vi "PH_SystemInformation.ProcCases.vi"(0 "i ref in":refnum<vi>, 1 "selector":string, 2 "Data":T1, 3 "call cluster":T2={"Object"="", "Selector"="", "CallType"=enum."synchronous", "Async Object"="", "Async Selector"="", "Data Descriptor"="", "Data"=[], "Error #"=0, "Expire"=0}, 5 "error in (no error)":errorcluster) -> (14 "i ref out":refnum<vi>, 17 "answer cluster":T2={"Object"="", "Selector"="", "CallType"=enum."synchronous", "Async Object"="", "Async Selector"="", "Data Descriptor"="", "Data"=[], "Error #"=0, "Expire"=0}, 19 "error out":errorcluster)   [LabVIEW 2014, in "PH_SystemInformation.lvlib"]
doc: "This method is called by a process from within the default case in the event loop. The methods of a class that are linked to events will be called from THIS method. Add your code here."
uses:
  PH_SystemInformation.lvlib
  CS_Core/CSSystem/CoreDefs/CoreDefs.call_type.ctl
  CS_Core/BaseProcess/BaseProcess.descriptor string definition.ctl
  CS_Core/CSSystem/CoreDefs/CoreDefs.rawDataType.ctl
  PH_SystemInformationEnabling State.ctl
  CS_Core/CSSystem/CoreLib/CoreLib.string 2 byte array.vi
  CS_Core/BaseProcess/BaseProcess.lvlib
  PH_Common/PH_Common.lvlib
  CS_Core/CAEObj/CAEObj.lvlib
  CS_Core/CSSystem/CoreLib/CoreLib.lvlib
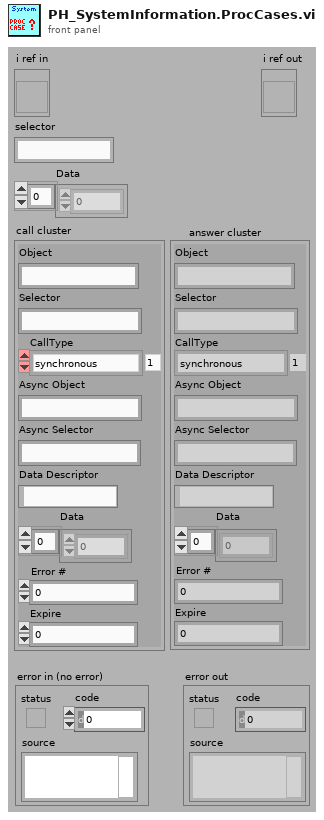
[diagram p1: front panel]
types:
  T1 = typedef "CoreDefs.rawDataType.ctl" = i8[]
  T2 = typedef "CoreDefs.call_type.ctl" = cluster{"Object":string, "Selector":string, "CallType":enum16{"simple", "synchronous", "asynchronous"}, "Async Object":string, "Async Selector":string, "Data Descriptor":T3, "Data":T1, "Error #":i32, "Expire":u32}
  T3 = typedef "BaseProcess.lvlib/BaseProcess.descriptor string definition.ctl" = string
  T4 = typedef "PH_SystemInformation.lvlib/PH_SystemInformation.i attribute.ctl" = cluster{"Laser Enabling":cluster{"GUI Ref":refnum<vi>, "Enabling State":T5}, "PreAmp Enabling":cluster{"GUI Ref":refnum<vi>, "Enabling State":T5}, "MainAmp Enabling":cluster{"GUI Ref":refnum<vi>, "Enabling State":T5}, "Emergency Off":cluster{"GUI Ref":refnum<vi>, "State":enum16{"no info", "off/false", "Alarm"}}, "Enabling Exp. 1":cluster{"GUI Ref":refnum<vi>, "Enabling State":T5}, "Enabling Exp. 2":cluster{"GUI Ref":refnum<vi>, "Enabling State":T5}, "Enabling Exp. 3":cluster{"GUI Ref":refnum<vi>, "Enabling State":T5}, "Enabling Exp. 4":cluster{"GUI Ref":refnum<vi>, "Enabling State":T5}, "Timing Mode":cluster{"GUI Ref":refnum<vi>, "PHELIX_Timing_Mode":enum32{"10 Hz", "0.5 Hz", "Shot"}}}
  T5 = typedef "PH_SystemInformation.lvlib/PH_SystemInformationEnabling State.ctl" = i32
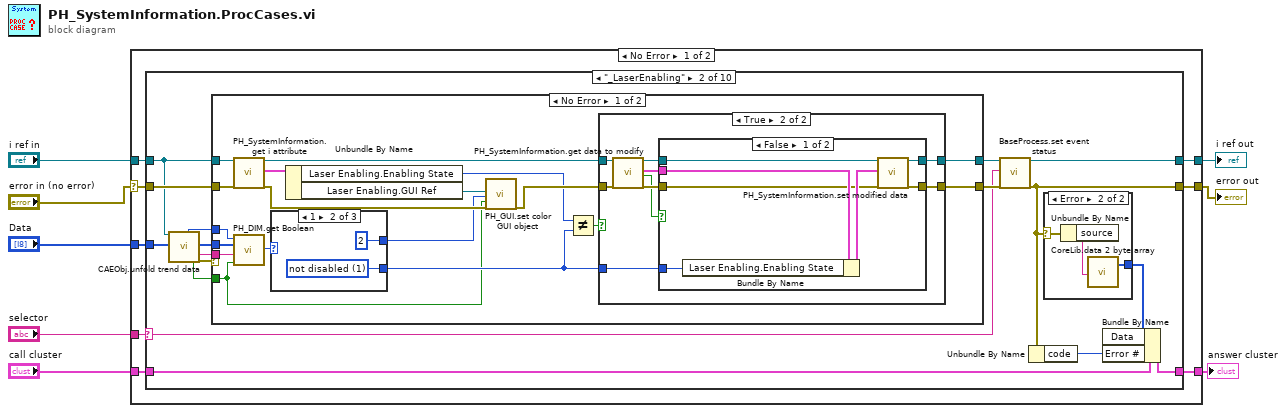
[diagram p0: block diagram]
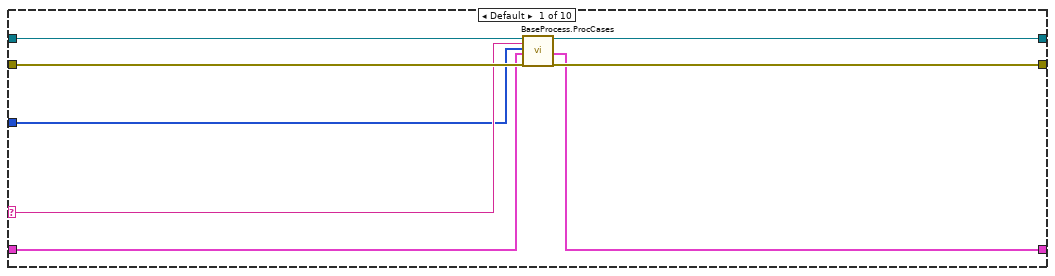
[diagram p2: hidden frame]
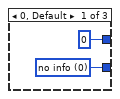
[diagram p6: hidden frame]
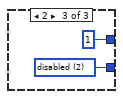
[diagram p7: hidden frame]
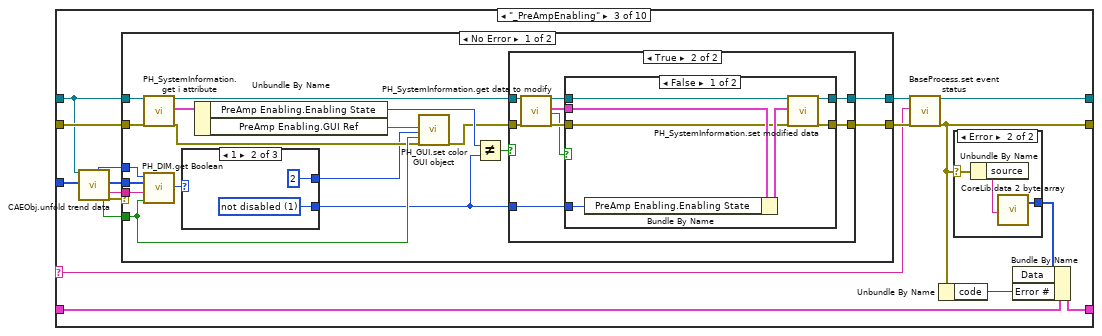
[diagram p9: hidden frame]
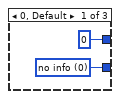
[diagram p13: hidden frame]
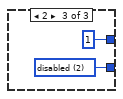
[diagram p14: hidden frame]
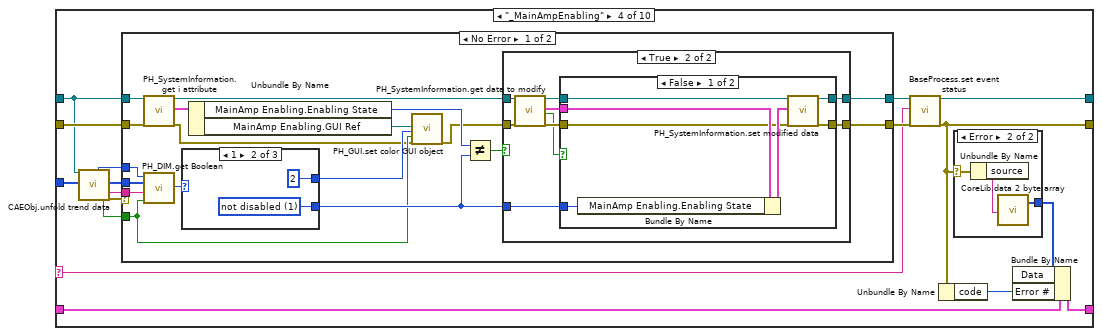
[diagram p16: hidden frame]
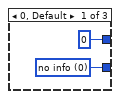
[diagram p20: hidden frame]
diagram:
  n1 = case shown="No Error" "error in (no error)" {
    selector: "error in (no error)" -> [w9 w624]
    tunnel: "selector" -> [w16 _]
    tunnel: [w15 w623] -> w7
    tunnel: "call cluster" -> [w14 w623]
    tunnel: "i ref in" -> [w13 w625]
    tunnel: [w12 w625] -> w4
    tunnel: [w11 w624] -> w3
    tunnel: "Data" -> [w10 _]
    frame No Error {
      n2 = case shown="\"_LaserEnabling\"" w16 {
        selector: w16 -> [w19 w27 w93 w159 w225 w291 w357 w423 w489 w555]
        tunnel: w10 -> [w17 w40 w106 w172 w238 w304 w370 w436 w502 w566]
        tunnel: w13 -> [w18 w39 w105 w171 w237 w303 w369 w435 w501 w565]
        tunnel: [w24 w28 w94 w160 w226 w292 w358 w424 w490 w556] -> w12
        tunnel: w14 -> [w20 w26 w92 w158 w224 w290 w356 w422 w488 w554]
        tunnel: [w21 w25 w91 w157 w223 w289 w355 w421 w487 w553] -> w15
        tunnel: w9 -> [w23 w41 w107 w173 w239 w305 w371 w437 w503 w567]
        tunnel: [w22 w29 w95 w161 w227 w293 w359 w425 w491 w557] -> w11
        frame Default {
          n3 = call "BaseProcess.ProcCases.vi"("i ref in"=w18, "selector"=w19, "Data"=w17, "call cluster"=w20, "error in (no error)"=w23) -> ("i ref out"=w24:refnum<vi>, "answer cluster"=w21:T2, "error out"=w22:errorcluster)  [unwired: 12 in]
        }
        frame "_LaserEnabling" {
          n4 = call "CAEObj.unfold trend data.vi"("i ref in"=w39, "raw trend data"=w40) -> ("quality"=w38:i32, "no link"=w36:bool, "data"=w35:i8[], "typeDescriptor"=w37:string, "error out"=w34:errorcluster)  [unwired: 9 in, 4 out]
          n5 = case shown="No Error" w34 {
            tunnel: [w57 w90] -> w30
            tunnel: w39 -> [w56 w90]
            tunnel: w41 -> [w62 w89]
            tunnel: [w58 w89] -> w31
            tunnel: w38 -> [w61 _]
            tunnel: w37 -> [w60 _]
            tunnel: w36 -> [w46 _]
            tunnel: w35 -> [w59 _]
            frame No Error {
              n6 = call "PH_SystemInformation.get i attribute.vi"("i ref in"=w56, "error in (no error)"=w62) -> ("i ref out"=w55:refnum<vi>, "i attribute"=w53:T4, "error out"=w50:errorcluster)  [unwired: 15 in]
              n7 = call "PH_DIM.get Boolean.vi"("no link"=w46, "typeDescriptor"=w60, "data"=w59, "quality"=w61) -> ("Value"=w54:i32)
              n8 = case shown="1" w54 {
                tunnel: [0 2 1] -> w47
                tunnel: [w83 w85 w87] -> w52
                frame 0, Default {
                  w83 = T5 0 items=["no info", "not disabled", "disabled"] ("Laser Enabling.Enabling State")
                }
                frame 1 {
                  w85 = T5 1 items=["no info", "not disabled", "disabled"] ("Laser Enabling.Enabling State")
                }
                frame 2 {
                  w87 = T5 2 items=["no info", "not disabled", "disabled"] ("Laser Enabling.Enabling State")
                }
              }
              n9 = Unbundle By Name(w53) -> ("Laser Enabling.Enabling State"=w45:T5, "Laser Enabling.GUI Ref"=w48:refnum<vi>)
              n10 = call "PH_GUI.set color GUI object.vi"("GUI object Ref"=w48, "State"=w47, "Blinking? (false)"=w46, "error in (no error)"=w50) -> ("error out"=w49:errorcluster)  [unwired: 15 in]
              n11 = Not Equal?(x=w45, y=w52) -> (x != y?=w51:bool)
              n12 = case shown="True" w51 {
                tunnel: [w63 w71] -> w58
                tunnel: [w64 w69] -> w57
                tunnel: w49 -> [w63 w67]
                tunnel: w55 -> [w64 w66]
                tunnel: w52 -> [_ w65]
                frame False {
                }
                frame True {
                  n13 = call "PH_SystemInformation.get data to modify.vi"("i ref in"=w66, "error in (no error)"=w67) -> ("i ref out"=w70:refnum<vi>, "i attribute"=w72:T4, "timed out"=w68:bool, "error out"=w73:errorcluster)  [unwired: 14 in]
                  n14 = case shown="False" w68 {
                    tunnel: w73 -> [w74 w81]
                    tunnel: w72 -> [w77 _]
                    tunnel: [w80 w81] -> w71
                    tunnel: w70 -> [w79 w82]
                    tunnel: [w78 w82] -> w69
                    tunnel: w65 -> [w75 _]
                    frame False {
                      n15 = Bundle By Name(cluster=w77, "Laser Enabling.Enabling State"=w75) -> (w76:T4)
                      n16 = call "PH_SystemInformation.set modified data.vi"("i ref in"=w79, "i attribute"=w76, "error in (no error)"=w74) -> ("i ref out"=w78:refnum<vi>, "error out"=w80:errorcluster)  [unwired: 15 in]
                    }
                    frame True {
                    }
                  }
                }
              }
            }
            frame Error {
            }
          }
          n17 = call "BaseProcess.set event status.vi"("i ref in"=w30, "EventStatus"=w27, "error in (no error)"=w31) -> ("i ref out"=w28:refnum<vi>, "error out"=w29:errorcluster)  [unwired: 14 in, 1 out]
          n18 = Unbundle By Name(w29) -> ("code"=w33:i32)
          n19 = case shown="Error" w29 {
            selector: w29 -> [_ w44]
            tunnel: [_ w42] -> w32
            frame No Error {
            }
            frame Error {
              n20 = Unbundle By Name(w44) -> ("source"=w43:string)
              n21 = call-poly "CoreLib.data 2 byte array.vi"("string"=w43) -> ("byteArray out"=w42:T1)  [unwired: 18 in]
            }
          }
          n22 = Bundle By Name(cluster=w26, "Data"=w32, "Error #"=w33) -> (w25:T2)
        }
        frame "_PreAmpEnabling" {
          n23 = call "CAEObj.unfold trend data.vi"("i ref in"=w105, "raw trend data"=w106) -> ("quality"=w104:i32, "no link"=w102:bool, "data"=w101:i8[], "typeDescriptor"=w103:string, "error out"=w100:errorcluster)  [unwired: 9 in, 4 out]
          n24 = case shown="No Error" w100 {
            tunnel: [w123 w156] -> w96
            tunnel: w105 -> [w122 w156]
            tunnel: w107 -> [w128 w155]
            tunnel: [w124 w155] -> w97
            tunnel: w104 -> [w127 _]
            tunnel: w103 -> [w126 _]
            tunnel: w102 -> [w115 _]
            tunnel: w101 -> [w125 _]
            frame No Error {
              n25 = call "PH_SystemInformation.get i attribute.vi"("i ref in"=w122, "error in (no error)"=w128) -> ("i ref out"=w121:refnum<vi>, "i attribute"=w119:T4, "error out"=w114:errorcluster)  [unwired: 15 in]
              n26 = call "PH_DIM.get Boolean.vi"("no link"=w115, "typeDescriptor"=w126, "data"=w125, "quality"=w127) -> ("Value"=w120:i32)
              n27 = case shown="1" w120 {
                tunnel: [0 2 1] -> w111
                tunnel: [w149 w151 w153] -> w112
                frame 0, Default {
                  w149 = T5 0 items=["no info", "not disabled", "disabled"] ("Laser Enabling.Enabling State")
                }
                frame 1 {
                  w151 = T5 1 items=["no info", "not disabled", "disabled"] ("Laser Enabling.Enabling State")
                }
                frame 2 {
                  w153 = T5 2 items=["no info", "not disabled", "disabled"] ("Laser Enabling.Enabling State")
                }
              }
              n28 = Unbundle By Name(w119) -> ("PreAmp Enabling.Enabling State"=w118:T5, "PreAmp Enabling.GUI Ref"=w116:refnum<vi>)
              n29 = call "PH_GUI.set color GUI object.vi"("GUI object Ref"=w116, "State"=w111, "Blinking? (false)"=w115, "error in (no error)"=w114) -> ("error out"=w113:errorcluster)  [unwired: 15 in]
              n30 = Not Equal?(x=w118, y=w112) -> (x != y?=w117:bool)
              n31 = case shown="True" w117 {
                tunnel: [w129 w137] -> w124
                tunnel: [w130 w135] -> w123
                tunnel: w113 -> [w129 w133]
                tunnel: w121 -> [w130 w132]
                tunnel: w112 -> [_ w131]
                frame False {
                }
                frame True {
                  n32 = call "PH_SystemInformation.get data to modify.vi"("i ref in"=w132, "error in (no error)"=w133) -> ("i ref out"=w136:refnum<vi>, "i attribute"=w138:T4, "timed out"=w134:bool, "error out"=w139:errorcluster)  [unwired: 14 in]
                  n33 = case shown="False" w134 {
                    tunnel: w139 -> [w140 w147]
                    tunnel: w138 -> [w143 _]
                    tunnel: [w146 w147] -> w137
                    tunnel: w136 -> [w145 w148]
                    tunnel: [w144 w148] -> w135
                    tunnel: w131 -> [w141 _]
                    frame False {
                      n34 = Bundle By Name(cluster=w143, "PreAmp Enabling.Enabling State"=w141) -> (w142:T4)
                      n35 = call "PH_SystemInformation.set modified data.vi"("i ref in"=w145, "i attribute"=w142, "error in (no error)"=w140) -> ("i ref out"=w144:refnum<vi>, "error out"=w146:errorcluster)  [unwired: 15 in]
                    }
                    frame True {
                    }
                  }
                }
              }
            }
            frame Error {
            }
          }
          n36 = call "BaseProcess.set event status.vi"("i ref in"=w96, "EventStatus"=w93, "error in (no error)"=w97) -> ("i ref out"=w94:refnum<vi>, "error out"=w95:errorcluster)  [unwired: 14 in, 1 out]
          n37 = Unbundle By Name(w95) -> ("code"=w99:i32)
          n38 = case shown="Error" w95 {
            selector: w95 -> [_ w110]
            tunnel: [_ w108] -> w98
            frame No Error {
            }
            frame Error {
              n39 = Unbundle By Name(w110) -> ("source"=w109:string)
              n40 = call-poly "CoreLib.data 2 byte array.vi"("string"=w109) -> ("byteArray out"=w108:T1)  [unwired: 18 in]
            }
          }
          n41 = Bundle By Name(cluster=w92, "Data"=w98, "Error #"=w99) -> (w91:T2)
        }
        frame "_MainAmpEnabling" {
          n42 = call "CAEObj.unfold trend data.vi"("i ref in"=w171, "raw trend data"=w172) -> ("quality"=w170:i32, "no link"=w168:bool, "data"=w167:i8[], "typeDescriptor"=w169:string, "error out"=w166:errorcluster)  [unwired: 9 in, 4 out]
          n43 = case shown="No Error" w166 {
            tunnel: [w189 w222] -> w162
            tunnel: w171 -> [w188 w222]
            tunnel: w173 -> [w194 w221]
            tunnel: [w190 w221] -> w163
            tunnel: w170 -> [w193 _]
            tunnel: w169 -> [w192 _]
            tunnel: w168 -> [w180 _]
            tunnel: w167 -> [w191 _]
            frame No Error {
              n44 = call "PH_SystemInformation.get i attribute.vi"("i ref in"=w188, "error in (no error)"=w194) -> ("i ref out"=w187:refnum<vi>, "i attribute"=w185:T4, "error out"=w178:errorcluster)  [unwired: 15 in]
              n45 = call "PH_DIM.get Boolean.vi"("no link"=w180, "typeDescriptor"=w192, "data"=w191, "quality"=w193) -> ("Value"=w186:i32)
              n46 = case shown="1" w186 {
                tunnel: [0 2 1] -> w181
                tunnel: [w215 w217 w219] -> w183
                frame 0, Default {
                  w215 = T5 0 items=["no info", "not disabled", "disabled"] ("Laser Enabling.Enabling State")
                }
                frame 1 {
                  w217 = T5 1 items=["no info", "not disabled", "disabled"] ("Laser Enabling.Enabling State")
                }
                frame 2 {
                  w219 = T5 2 items=["no info", "not disabled", "disabled"] ("Laser Enabling.Enabling State")
                }
              }
              n47 = Unbundle By Name(w185) -> ("MainAmp Enabling.Enabling State"=w184:T5, "MainAmp Enabling.GUI Ref"=w177:refnum<vi>)
              n48 = call "PH_GUI.set color GUI object.vi"("GUI object Ref"=w177, "State"=w181, "Blinking? (false)"=w180, "error in (no error)"=w178) -> ("error out"=w179:errorcluster)  [unwired: 15 in]
              n49 = Not Equal?(x=w184, y=w183) -> (x != y?=w182:bool)
              n50 = case shown="True" w182 {
                tunnel: [w195 w203] -> w190
                tunnel: [w196 w201] -> w189
                tunnel: w179 -> [w195 w199]
                tunnel: w187 -> [w196 w198]
                tunnel: w183 -> [_ w197]
                frame False {
                }
                frame True {
                  n51 = call "PH_SystemInformation.get data to modify.vi"("i ref in"=w198, "error in (no error)"=w199) -> ("i ref out"=w202:refnum<vi>, "i attribute"=w204:T4, "timed out"=w200:bool, "error out"=w205:errorcluster)  [unwired: 14 in]
                  n52 = case shown="False" w200 {
                    tunnel: w205 -> [w206 w213]
                    tunnel: w204 -> [w209 _]
                    tunnel: [w212 w213] -> w203
                    tunnel: w202 -> [w211 w214]
                    tunnel: [w210 w214] -> w201
                    tunnel: w197 -> [w207 _]
                    frame False {
                      n53 = Bundle By Name(cluster=w209, "MainAmp Enabling.Enabling State"=w207) -> (w208:T4)
                      n54 = call "PH_SystemInformation.set modified data.vi"("i ref in"=w211, "i attribute"=w208, "error in (no error)"=w206) -> ("i ref out"=w210:refnum<vi>, "error out"=w212:errorcluster)  [unwired: 15 in]
                    }
                    frame True {
                    }
                  }
                }
              }
            }
            frame Error {
            }
          }
          n55 = call "BaseProcess.set event status.vi"("i ref in"=w162, "EventStatus"=w159, "error in (no error)"=w163) -> ("i ref out"=w160:refnum<vi>, "error out"=w161:errorcluster)  [unwired: 14 in, 1 out]
          n56 = Unbundle By Name(w161) -> ("code"=w165:i32)
          n57 = case shown="Error" w161 {
            selector: w161 -> [_ w176]
            tunnel: [_ w174] -> w164
            frame No Error {
            }
            frame Error {
              n58 = Unbundle By Name(w176) -> ("source"=w175:string)
              n59 = call-poly "CoreLib.data 2 byte array.vi"("string"=w175) -> ("byteArray out"=w174:T1)  [unwired: 18 in]
            }
          }
          n60 = Bundle By Name(cluster=w158, "Data"=w164, "Error #"=w165) -> (w157:T2)
        }
        frame "_EmergencyOff" {
          n61 = call "CAEObj.unfold trend data.vi"("i ref in"=w237, "raw trend data"=w238) -> ("quality"=w236:i32, "no link"=w234:bool, "data"=w233:i8[], "typeDescriptor"=w235:string, "error out"=w232:errorcluster)  [unwired: 9 in, 4 out]
          n62 = case shown="No Error" w232 {
            tunnel: [w255 w288] -> w228
            tunnel: w237 -> [w254 w288]
            tunnel: w239 -> [w260 w287]
            tunnel: [w256 w287] -> w229
            tunnel: w236 -> [w259 _]
            tunnel: w235 -> [w258 _]
            tunnel: w234 -> [w245 _]
            tunnel: w233 -> [w257 _]
            frame No Error {
              n63 = call "PH_SystemInformation.get i attribute.vi"("i ref in"=w254, "error in (no error)"=w260) -> ("i ref out"=w253:refnum<vi>, "i attribute"=w252:T4, "error out"=w244:errorcluster)  [unwired: 15 in]
              n64 = call "PH_DIM.get Boolean.vi"("no link"=w245, "typeDescriptor"=w258, "data"=w257, "quality"=w259) -> ("Value"=w249:i32)
              n65 = case shown="1" w249 {
                tunnel: [0 1 4] -> w246
                tunnel: [enum16{"no info", "off/false", "Alarm"}."no info" ("Emergency Off.State") enum16{"no info", "off/false", "Alarm"}."off/false" ("Emergency Off.State") enum16{"no info", "off/false", "Alarm"}."Alarm" ("Emergency Off.State")] -> w248
                frame 0, Default {
                }
                frame 1 {
                }
                frame 2 {
                }
              }
              n66 = Unbundle By Name(w252) -> ("Emergency Off.State"=w251:enum16{"no info", "off/false", "Alarm"}, "Emergency Off.GUI Ref"=w247:refnum<vi>)
              n67 = call "PH_GUI.set color GUI object.vi"("GUI object Ref"=w247, "State"=w246, "Blinking? (false)"=w245, "error in (no error)"=w244) -> ("error out"=w243:errorcluster)  [unwired: 15 in]
              n68 = Not Equal?(x=w251, y=w248) -> (x != y?=w250:bool)
              n69 = case shown="True" w250 {
                tunnel: [w267 w275] -> w256
                tunnel: [w268 w273] -> w255
                tunnel: w243 -> [w267 w271]
                tunnel: w253 -> [w268 w270]
                tunnel: w248 -> [_ w269]
                frame False {
                }
                frame True {
                  n70 = call "PH_SystemInformation.get data to modify.vi"("i ref in"=w270, "error in (no error)"=w271) -> ("i ref out"=w274:refnum<vi>, "i attribute"=w276:T4, "timed out"=w272:bool, "error out"=w277:errorcluster)  [unwired: 14 in]
                  n71 = case shown="False" w272 {
                    tunnel: w277 -> [w278 w285]
                    tunnel: w276 -> [w281 _]
                    tunnel: [w284 w285] -> w275
                    tunnel: w274 -> [w283 w286]
                    tunnel: [w282 w286] -> w273
                    tunnel: w269 -> [w279 _]
                    frame False {
                      n72 = Bundle By Name(cluster=w281, "Emergency Off.State"=w279) -> (w280:T4)
                      n73 = call "PH_SystemInformation.set modified data.vi"("i ref in"=w283, "i attribute"=w280, "error in (no error)"=w278) -> ("i ref out"=w282:refnum<vi>, "error out"=w284:errorcluster)  [unwired: 15 in]
                    }
                    frame True {
                    }
                  }
                }
              }
            }
            frame Error {
            }
          }
          n74 = call "BaseProcess.set event status.vi"("i ref in"=w228, "EventStatus"=w225, "error in (no error)"=w229) -> ("i ref out"=w226:refnum<vi>, "error out"=w227:errorcluster)  [unwired: 14 in, 1 out]
          n75 = Unbundle By Name(w227) -> ("code"=w231:i32)
          n76 = case shown="Error" w227 {
            selector: w227 -> [_ w242]
            tunnel: [_ w240] -> w230
            frame No Error {
            }
            frame Error {
              n77 = Unbundle By Name(w242) -> ("source"=w241:string)
              n78 = call-poly "CoreLib.data 2 byte array.vi"("string"=w241) -> ("byteArray out"=w240:T1)  [unwired: 18 in]
            }
          }
          n79 = Bundle By Name(cluster=w224, "Data"=w230, "Error #"=w231) -> (w223:T2)
        }
        frame "_Exp1Enabling" {
          n80 = call "CAEObj.unfold trend data.vi"("i ref in"=w303, "raw trend data"=w304) -> ("quality"=w302:i32, "no link"=w300:bool, "data"=w299:i8[], "typeDescriptor"=w301:string, "error out"=w298:errorcluster)  [unwired: 9 in, 4 out]
          n81 = case shown="No Error" w298 {
            tunnel: [w321 w354] -> w294
            tunnel: w303 -> [w320 w354]
            tunnel: w305 -> [w326 w353]
            tunnel: [w322 w353] -> w295
            tunnel: w302 -> [w325 _]
            tunnel: w301 -> [w324 _]
            tunnel: w300 -> [w309 _]
            tunnel: w299 -> [w323 _]
            frame No Error {
              n82 = call "PH_SystemInformation.get i attribute.vi"("i ref in"=w320, "error in (no error)"=w326) -> ("i ref out"=w319:refnum<vi>, "i attribute"=w318:T4, "error out"=w313:errorcluster)  [unwired: 15 in]
              n83 = call "PH_DIM.get Boolean.vi"("no link"=w309, "typeDescriptor"=w324, "data"=w323, "quality"=w325) -> ("Value"=w315:i32)
              n84 = case shown="2" w315 {
                tunnel: [0 2 1] -> w310
                tunnel: [w327 w329 w331] -> w314
                frame 0, Default {
                  w327 = T5 0 items=["no info", "not disabled", "disabled"] ("Laser Enabling.Enabling State")
                }
                frame 1 {
                  w329 = T5 1 items=["no info", "not disabled", "disabled"] ("Laser Enabling.Enabling State")
                }
                frame 2 {
                  w331 = T5 2 items=["no info", "not disabled", "disabled"] ("Laser Enabling.Enabling State")
                }
              }
              n85 = Unbundle By Name(w318) -> ("Enabling Exp. 1.Enabling State"=w317:T5, "Enabling Exp. 1.GUI Ref"=w311:refnum<vi>)
              n86 = call "PH_GUI.set color GUI object.vi"("GUI object Ref"=w311, "State"=w310, "Blinking? (false)"=w309, "error in (no error)"=w313) -> ("error out"=w312:errorcluster)  [unwired: 15 in]
              n87 = Not Equal?(x=w317, y=w314) -> (x != y?=w316:bool)
              n88 = case shown="True" w316 {
                tunnel: [w333 w341] -> w322
                tunnel: [w334 w339] -> w321
                tunnel: w312 -> [w333 w337]
                tunnel: w319 -> [w334 w336]
                tunnel: w314 -> [_ w335]
                frame False {
                }
                frame True {
                  n89 = call "PH_SystemInformation.get data to modify.vi"("i ref in"=w336, "error in (no error)"=w337) -> ("i ref out"=w340:refnum<vi>, "i attribute"=w342:T4, "timed out"=w338:bool, "error out"=w343:errorcluster)  [unwired: 14 in]
                  n90 = case shown="False" w338 {
                    tunnel: w343 -> [w344 w351]
                    tunnel: w342 -> [w347 _]
                    tunnel: [w350 w351] -> w341
                    tunnel: w340 -> [w349 w352]
                    tunnel: [w348 w352] -> w339
                    tunnel: w335 -> [w345 _]
                    frame False {
                      n91 = Bundle By Name(cluster=w347, "Enabling Exp. 1.Enabling State"=w345) -> (w346:T4)
                      n92 = call "PH_SystemInformation.set modified data.vi"("i ref in"=w349, "i attribute"=w346, "error in (no error)"=w344) -> ("i ref out"=w348:refnum<vi>, "error out"=w350:errorcluster)  [unwired: 15 in]
                    }
                    frame True {
                    }
                  }
                }
              }
            }
            frame Error {
            }
          }
          n93 = call "BaseProcess.set event status.vi"("i ref in"=w294, "EventStatus"=w291, "error in (no error)"=w295) -> ("i ref out"=w292:refnum<vi>, "error out"=w293:errorcluster)  [unwired: 14 in, 1 out]
          n94 = Unbundle By Name(w293) -> ("code"=w297:i32)
          n95 = case shown="Error" w293 {
            selector: w293 -> [_ w308]
            tunnel: [_ w306] -> w296
            frame No Error {
            }
            frame Error {
              n96 = Unbundle By Name(w308) -> ("source"=w307:string)
              n97 = call-poly "CoreLib.data 2 byte array.vi"("string"=w307) -> ("byteArray out"=w306:T1)  [unwired: 18 in]
            }
          }
          n98 = Bundle By Name(cluster=w290, "Data"=w296, "Error #"=w297) -> (w289:T2)
        }
        frame "_Exp2Enabling" {
          n99 = call "CAEObj.unfold trend data.vi"("i ref in"=w369, "raw trend data"=w370) -> ("quality"=w368:i32, "no link"=w366:bool, "data"=w365:i8[], "typeDescriptor"=w367:string, "error out"=w364:errorcluster)  [unwired: 9 in, 4 out]
          n100 = case shown="No Error" w364 {
            tunnel: [w387 w420] -> w360
            tunnel: w369 -> [w386 w420]
            tunnel: w371 -> [w392 w419]
            tunnel: [w388 w419] -> w361
            tunnel: w368 -> [w391 _]
            tunnel: w367 -> [w390 _]
            tunnel: w366 -> [w378 _]
            tunnel: w365 -> [w389 _]
            frame No Error {
              n101 = call "PH_SystemInformation.get i attribute.vi"("i ref in"=w386, "error in (no error)"=w392) -> ("i ref out"=w385:refnum<vi>, "i attribute"=w384:T4, "error out"=w376:errorcluster)  [unwired: 15 in]
              n102 = call "PH_DIM.get Boolean.vi"("no link"=w378, "typeDescriptor"=w390, "data"=w389, "quality"=w391) -> ("Value"=w381:i32)
              n103 = case shown="2" w381 {
                tunnel: [0 2 1] -> w379
                tunnel: [w393 w395 w397] -> w380
                frame 0, Default {
                  w393 = T5 0 items=["no info", "not disabled", "disabled"] ("Laser Enabling.Enabling State")
                }
                frame 1 {
                  w395 = T5 1 items=["no info", "not disabled", "disabled"] ("Laser Enabling.Enabling State")
                }
                frame 2 {
                  w397 = T5 2 items=["no info", "not disabled", "disabled"] ("Laser Enabling.Enabling State")
                }
              }
              n104 = Unbundle By Name(w384) -> ("Enabling Exp. 2.Enabling State"=w383:T5, "Enabling Exp. 2.GUI Ref"=w377:refnum<vi>)
              n105 = call "PH_GUI.set color GUI object.vi"("GUI object Ref"=w377, "State"=w379, "Blinking? (false)"=w378, "error in (no error)"=w376) -> ("error out"=w375:errorcluster)  [unwired: 15 in]
              n106 = Not Equal?(x=w383, y=w380) -> (x != y?=w382:bool)
              n107 = case shown="True" w382 {
                tunnel: [w399 w407] -> w388
                tunnel: [w400 w405] -> w387
                tunnel: w375 -> [w399 w403]
                tunnel: w385 -> [w400 w402]
                tunnel: w380 -> [_ w401]
                frame False {
                }
                frame True {
                  n108 = call "PH_SystemInformation.get data to modify.vi"("i ref in"=w402, "error in (no error)"=w403) -> ("i ref out"=w406:refnum<vi>, "i attribute"=w408:T4, "timed out"=w404:bool, "error out"=w409:errorcluster)  [unwired: 14 in]
                  n109 = case shown="False" w404 {
                    tunnel: w409 -> [w410 w417]
                    tunnel: w408 -> [w413 _]
                    tunnel: [w416 w417] -> w407
                    tunnel: w406 -> [w415 w418]
                    tunnel: [w414 w418] -> w405
                    tunnel: w401 -> [w411 _]
                    frame False {
                      n110 = Bundle By Name(cluster=w413, "Enabling Exp. 2.Enabling State"=w411) -> (w412:T4)
                      n111 = call "PH_SystemInformation.set modified data.vi"("i ref in"=w415, "i attribute"=w412, "error in (no error)"=w410) -> ("i ref out"=w414:refnum<vi>, "error out"=w416:errorcluster)  [unwired: 15 in]
                    }
                    frame True {
                    }
                  }
                }
              }
            }
            frame Error {
            }
          }
          n112 = call "BaseProcess.set event status.vi"("i ref in"=w360, "EventStatus"=w357, "error in (no error)"=w361) -> ("i ref out"=w358:refnum<vi>, "error out"=w359:errorcluster)  [unwired: 14 in, 1 out]
          n113 = Unbundle By Name(w359) -> ("code"=w363:i32)
          n114 = case shown="Error" w359 {
            selector: w359 -> [_ w374]
            tunnel: [_ w372] -> w362
            frame No Error {
            }
            frame Error {
              n115 = Unbundle By Name(w374) -> ("source"=w373:string)
              n116 = call-poly "CoreLib.data 2 byte array.vi"("string"=w373) -> ("byteArray out"=w372:T1)  [unwired: 18 in]
            }
          }
          n117 = Bundle By Name(cluster=w356, "Data"=w362, "Error #"=w363) -> (w355:T2)
        }
        frame "_Exp3Enabling" {
          n118 = call "CAEObj.unfold trend data.vi"("i ref in"=w435, "raw trend data"=w436) -> ("quality"=w434:i32, "no link"=w432:bool, "data"=w431:i8[], "typeDescriptor"=w433:string, "error out"=w430:errorcluster)  [unwired: 9 in, 4 out]
          n119 = case shown="No Error" w430 {
            tunnel: [w453 w486] -> w426
            tunnel: w435 -> [w452 w486]
            tunnel: w437 -> [w458 w485]
            tunnel: [w454 w485] -> w427
            tunnel: w434 -> [w457 _]
            tunnel: w433 -> [w456 _]
            tunnel: w432 -> [w442 _]
            tunnel: w431 -> [w455 _]
            frame No Error {
              n120 = call "PH_SystemInformation.get i attribute.vi"("i ref in"=w452, "error in (no error)"=w458) -> ("i ref out"=w451:refnum<vi>, "i attribute"=w450:T4, "error out"=w445:errorcluster)  [unwired: 15 in]
              n121 = call "PH_DIM.get Boolean.vi"("no link"=w442, "typeDescriptor"=w456, "data"=w455, "quality"=w457) -> ("Value"=w447:i32)
              n122 = case shown="2" w447 {
                tunnel: [0 2 1] -> w443
                tunnel: [w459 w461 w463] -> w446
                frame 0, Default {
                  w459 = T5 0 items=["no info", "not disabled", "disabled"] ("Laser Enabling.Enabling State")
                }
                frame 1 {
                  w461 = T5 1 items=["no info", "not disabled", "disabled"] ("Laser Enabling.Enabling State")
                }
                frame 2 {
                  w463 = T5 2 items=["no info", "not disabled", "disabled"] ("Laser Enabling.Enabling State")
                }
              }
              n123 = Unbundle By Name(w450) -> ("Enabling Exp. 3.Enabling State"=w449:T5, "Enabling Exp. 3.GUI Ref"=w441:refnum<vi>)
              n124 = call "PH_GUI.set color GUI object.vi"("GUI object Ref"=w441, "State"=w443, "Blinking? (false)"=w442, "error in (no error)"=w445) -> ("error out"=w444:errorcluster)  [unwired: 15 in]
              n125 = Not Equal?(x=w449, y=w446) -> (x != y?=w448:bool)
              n126 = case shown="True" w448 {
                tunnel: [w465 w473] -> w454
                tunnel: [w466 w471] -> w453
                tunnel: w444 -> [w465 w469]
                tunnel: w451 -> [w466 w468]
                tunnel: w446 -> [_ w467]
                frame False {
                }
                frame True {
                  n127 = call "PH_SystemInformation.get data to modify.vi"("i ref in"=w468, "error in (no error)"=w469) -> ("i ref out"=w472:refnum<vi>, "i attribute"=w474:T4, "timed out"=w470:bool, "error out"=w475:errorcluster)  [unwired: 14 in]
                  n128 = case shown="False" w470 {
                    tunnel: w475 -> [w476 w483]
                    tunnel: w474 -> [w479 _]
                    tunnel: [w482 w483] -> w473
                    tunnel: w472 -> [w481 w484]
                    tunnel: [w480 w484] -> w471
                    tunnel: w467 -> [w477 _]
                    frame False {
                      n129 = Bundle By Name(cluster=w479, "Enabling Exp. 3.Enabling State"=w477) -> (w478:T4)
                      n130 = call "PH_SystemInformation.set modified data.vi"("i ref in"=w481, "i attribute"=w478, "error in (no error)"=w476) -> ("i ref out"=w480:refnum<vi>, "error out"=w482:errorcluster)  [unwired: 15 in]
                    }
                    frame True {
                    }
                  }
                }
              }
            }
            frame Error {
            }
          }
          n131 = call "BaseProcess.set event status.vi"("i ref in"=w426, "EventStatus"=w423, "error in (no error)"=w427) -> ("i ref out"=w424:refnum<vi>, "error out"=w425:errorcluster)  [unwired: 14 in, 1 out]
          n132 = Unbundle By Name(w425) -> ("code"=w429:i32)
          n133 = case shown="Error" w425 {
            selector: w425 -> [_ w440]
            tunnel: [_ w438] -> w428
            frame No Error {
            }
            frame Error {
              n134 = Unbundle By Name(w440) -> ("source"=w439:string)
              n135 = call-poly "CoreLib.data 2 byte array.vi"("string"=w439) -> ("byteArray out"=w438:T1)  [unwired: 18 in]
            }
          }
          n136 = Bundle By Name(cluster=w422, "Data"=w428, "Error #"=w429) -> (w421:T2)
        }
        frame "_Exp4Enabling" {
          n137 = call "CAEObj.unfold trend data.vi"("i ref in"=w501, "raw trend data"=w502) -> ("quality"=w500:i32, "no link"=w498:bool, "data"=w497:i8[], "typeDescriptor"=w499:string, "error out"=w496:errorcluster)  [unwired: 9 in, 4 out]
          n138 = case shown="No Error" w496 {
            tunnel: [w519 w552] -> w492
            tunnel: w501 -> [w518 w552]
            tunnel: w503 -> [w524 w551]
            tunnel: [w520 w551] -> w493
            tunnel: w500 -> [w523 _]
            tunnel: w499 -> [w522 _]
            tunnel: w498 -> [w510 _]
            tunnel: w497 -> [w521 _]
            frame No Error {
              n139 = call "PH_SystemInformation.get i attribute.vi"("i ref in"=w518, "error in (no error)"=w524) -> ("i ref out"=w517:refnum<vi>, "i attribute"=w516:T4, "error out"=w509:errorcluster)  [unwired: 15 in]
              n140 = call "PH_DIM.get Boolean.vi"("no link"=w510, "typeDescriptor"=w522, "data"=w521, "quality"=w523) -> ("Value"=w513:i32)
              n141 = case shown="2" w513 {
                tunnel: [0 2 1] -> w511
                tunnel: [w525 w527 w529] -> w512
                frame 0, Default {
                  w525 = T5 0 items=["no info", "not disabled", "disabled"] ("Laser Enabling.Enabling State")
                }
                frame 1 {
                  w527 = T5 1 items=["no info", "not disabled", "disabled"] ("Laser Enabling.Enabling State")
                }
                frame 2 {
                  w529 = T5 2 items=["no info", "not disabled", "disabled"] ("Laser Enabling.Enabling State")
                }
              }
              n142 = Unbundle By Name(w516) -> ("Enabling Exp. 4.Enabling State"=w515:T5, "Enabling Exp. 4.GUI Ref"=w507:refnum<vi>)
              n143 = call "PH_GUI.set color GUI object.vi"("GUI object Ref"=w507, "State"=w511, "Blinking? (false)"=w510, "error in (no error)"=w509) -> ("error out"=w508:errorcluster)  [unwired: 15 in]
              n144 = Not Equal?(x=w515, y=w512) -> (x != y?=w514:bool)
              n145 = case shown="True" w514 {
                tunnel: [w531 w539] -> w520
                tunnel: [w532 w537] -> w519
                tunnel: w508 -> [w531 w535]
                tunnel: w517 -> [w532 w534]
                tunnel: w512 -> [_ w533]
                frame False {
                }
                frame True {
                  n146 = call "PH_SystemInformation.get data to modify.vi"("i ref in"=w534, "error in (no error)"=w535) -> ("i ref out"=w538:refnum<vi>, "i attribute"=w540:T4, "timed out"=w536:bool, "error out"=w541:errorcluster)  [unwired: 14 in]
                  n147 = case shown="False" w536 {
                    tunnel: w541 -> [w542 w549]
                    tunnel: w540 -> [w545 _]
                    tunnel: [w548 w549] -> w539
                    tunnel: w538 -> [w547 w550]
                    tunnel: [w546 w550] -> w537
                    tunnel: w533 -> [w543 _]
                    frame False {
                      n148 = Bundle By Name(cluster=w545, "Enabling Exp. 4.Enabling State"=w543) -> (w544:T4)
                      n149 = call "PH_SystemInformation.set modified data.vi"("i ref in"=w547, "i attribute"=w544, "error in (no error)"=w542) -> ("i ref out"=w546:refnum<vi>, "error out"=w548:errorcluster)  [unwired: 15 in]
                    }
                    frame True {
                    }
                  }
                }
              }
            }
            frame Error {
            }
          }
          n150 = call "BaseProcess.set event status.vi"("i ref in"=w492, "EventStatus"=w489, "error in (no error)"=w493) -> ("i ref out"=w490:refnum<vi>, "error out"=w491:errorcluster)  [unwired: 14 in, 1 out]
          n151 = Unbundle By Name(w491) -> ("code"=w495:i32)
          n152 = case shown="Error" w491 {
            selector: w491 -> [_ w506]
            tunnel: [_ w504] -> w494
            frame No Error {
            }
            frame Error {
              n153 = Unbundle By Name(w506) -> ("source"=w505:string)
              n154 = call-poly "CoreLib.data 2 byte array.vi"("string"=w505) -> ("byteArray out"=w504:T1)  [unwired: 18 in]
            }
          }
          n155 = Bundle By Name(cluster=w488, "Data"=w494, "Error #"=w495) -> (w487:T2)
        }
        frame "_TimingMode" {
          n156 = call "CAEObj.unfold trend data.vi"("i ref in"=w565, "raw trend data"=w566) -> ("no link"=w564:bool, "data"=w563:i8[], "error out"=w562:errorcluster)  [unwired: 9 in, 6 out]
          n157 = case shown="No Error" w562 {
            tunnel: [w590 w622] -> w558
            tunnel: w565 -> [w581 w622]
            tunnel: w567 -> [w582 w621]
            tunnel: [w591 w621] -> w559
            tunnel: w564 -> [w583 _]
            tunnel: w563 -> [w584 _]
            frame No Error {
              n158 = call "PH_SystemInformation.get i attribute.vi"("i ref in"=w581, "error in (no error)"=w582) -> ("i ref out"=w580:refnum<vi>, "i attribute"=w579:T4, "error out"=w574:errorcluster)  [unwired: 15 in]
              n159 = Type Cast(type=i16 0, x=w584) -> (*(type *) &x=w585:i16)
              n160 = Unbundle By Name(w579) -> ("Timing Mode.PHELIX_Timing_Mode"=w573:enum32{"10 Hz", "0.5 Hz", "Shot"}, "Timing Mode.GUI Ref"=w575:refnum<vi>)
              n161 = Equal?(x=i16 -1, y=w585) -> (x = y?=w587:bool)
              n162 = case shown="2" w585 {
                tunnel: [enum32{"10 Hz", "0.5 Hz", "Shot"}."10 Hz" ("Timing Mode.PHELIX_Timing_Mode") enum32{"10 Hz", "0.5 Hz", "Shot"}."0.5 Hz" ("Timing Mode.PHELIX_Timing_Mode") enum32{"10 Hz", "0.5 Hz", "Shot"}."Shot" ("Timing Mode.PHELIX_Timing_Mode")] -> w572
                frame 0, Default {
                }
                frame 1 {
                }
                frame 2 {
                }
              }
              n163 = Select(t=TRUE, s=w587, f=w583) -> (s? t:f=w577:bool)
              n164 = Not Equal?(x=w573, y=w572) -> (x != y?=w571:bool)
              n165 = Not A Number/Path/Refnum?(number/path/refnum=w575) -> (NaN/Path/Refnum?=w578:bool)
              n166 = case shown="False" w578 {
                tunnel: w574 -> [w616 w617]
                tunnel: [w615 w617] -> w576
                tunnel: w575 -> [w614 _]
                tunnel: w572 -> [w613 _]
                tunnel: w577 -> [w612 _]
                frame False {
                  n167 = property class="RadioBtnsControl (strict)"(reference=w614, error in=w616, "Value"=w613, "Blinking"=w612) -> (error out=w615:errorcluster)  [unwired: 1 out]
                }
                frame True {
                }
              }
              n168 = case shown="True" w571 {
                tunnel: [w592 w600] -> w591
                tunnel: [w593 w598] -> w590
                tunnel: w580 -> [w593 w596]
                tunnel: w572 -> [_ w595]
                tunnel: w576 -> [w592 w594]
                frame False {
                }
                frame True {
                  n169 = call "PH_SystemInformation.get data to modify.vi"("i ref in"=w596, "error in (no error)"=w594) -> ("i ref out"=w599:refnum<vi>, "i attribute"=w601:T4, "timed out"=w597:bool, "error out"=w602:errorcluster)  [unwired: 14 in]
                  n170 = case shown="False" w597 {
                    tunnel: w602 -> [w603 w610]
                    tunnel: w601 -> [w606 _]
                    tunnel: [w609 w610] -> w600
                    tunnel: w599 -> [w608 w611]
                    tunnel: [w607 w611] -> w598
                    tunnel: w595 -> [w604 _]
                    frame False {
                      n171 = Bundle By Name(cluster=w606, "Timing Mode.PHELIX_Timing_Mode"=w604) -> (w605:T4)
                      n172 = call "PH_SystemInformation.set modified data.vi"("i ref in"=w608, "i attribute"=w605, "error in (no error)"=w603) -> ("i ref out"=w607:refnum<vi>, "error out"=w609:errorcluster)  [unwired: 15 in]
                    }
                    frame True {
                    }
                  }
                }
              }
            }
            frame Error {
            }
          }
          n173 = call "BaseProcess.set event status.vi"("i ref in"=w558, "EventStatus"=w555, "error in (no error)"=w559) -> ("i ref out"=w556:refnum<vi>, "error out"=w557:errorcluster)  [unwired: 14 in, 1 out]
          n174 = Unbundle By Name(w557) -> ("code"=w561:i32)
          n175 = case shown="Error" w557 {
            selector: w557 -> [_ w570]
            tunnel: [_ w568] -> w560
            frame No Error {
            }
            frame Error {
              n176 = Unbundle By Name(w570) -> ("source"=w569:string)
              n177 = call-poly "CoreLib.data 2 byte array.vi"("string"=w569) -> ("byteArray out"=w568:T1)  [unwired: 18 in]
            }
          }
          n178 = Bundle By Name(cluster=w554, "Data"=w560, "Error #"=w561) -> (w553:T2)
        }
      }
    }
    frame Error {
    }
  }
  "answer cluster" <- w7
  "i ref out" <- w4
  "error out" <- w3
